vi "Aux CO2 Serial Close.vi"(8 "error in":errorcluster, 10 "Capno Data In":T1={"Port"="", "Source"=0, "Active"=FALSE, "Baro Pressure"=760, "SerialRxBuffer"="", "Raw CO2 (Torr)"=5.0, "bytes read"=5, "Status"=[], "Status Message"=enum.""} {"Status" format="%x"; "Baro Pressure" min=400 max=800; "Source" items=["None", "TidalWave", "LoFlow / Canary", "Capnogard"]}, 11 "Serial Port In":T3={"termination char"=10, "End read on termination character?"=TRUE, "Enabled?"=FALSE, "VISA resource name"="COM1", "baud rate"=9600, "data bits"=8, "parity"=enum."None", "stop bits"=10, "flow control"=0, "timeout (ms)"=10000, "Input buffer size"=4096, "End write on termination character?"=TRUE, "XON Char"=17, "XOFF Char"=19} {"XOFF Char" format="%.0x"; "XON Char" format="%.0x"; "flow control" items=["None"=0, "XON/XOFF"=1, "RTS/CTS"=2, "DTR/DSR"=4]; "stop bits" items=["1.0"=10, "1.5"=15, "2.0"=20]; "data bits" min=5 max=8 step=1; "baud rate" items=["75"=75, "110"=110, "134"=134, "150"=150, "300"=300, "600"=600, "1200"=1200, "1800"=1800, "2400"=2400, "4800"=4800, "7200"=7200, "9600"=9600, "14400"=14400, "19200"=19200, "28800"=28800, "38400"=38400, "56000"=56000, "57600"=57600, "115200"=115200, "128000"=128000, "230400"=230400]; "termination char" format="%.0x"}) -> (0 "error out":errorcluster, 2 "Capno Data Out":T1={"Port"="", "Source"=0, "Active"=FALSE, "Baro Pressure"=760, "SerialRxBuffer"="", "Raw CO2 (Torr)"=5.0, "bytes read"=5, "Status"=[], "Status Message"=enum.""} {"Status" format="%x"; "Baro Pressure" min=400 max=800; "Source" items=["None", "TidalWave", "LoFlow / Canary", "Capnogard"]}, 3 "Serial Port Out":T3={"termination char"=10, "End read on termination character?"=TRUE, "Enabled?"=TRUE, "VISA resource name"="COM1", "baud rate"=9600, "data bits"=8, "parity"=enum."None", "stop bits"=10, "flow control"=0, "timeout (ms)"=10000, "Input buffer size"=4096, "End write on termination character?"=FALSE, "XON Char"=17, "XOFF Char"=19} {"XOFF Char" format="%.0x"; "XON Char" format="%.0x"; "flow control" items=["None"=0, "XON/XOFF"=1, "RTS/CTS"=2, "DTR/DSR"=4]; "stop bits" items=["1.0"=10, "1.5"=15, "2.0"=20]; "baud rate" items=["1.0"=10, "1.5"=15, "2.0"=20]; "termination char" format="%.0x"})   [LabVIEW 2016]
uses:
  Controls/Serial Visa Control.ctl
  Controls/Aux CO2 Diags.ctl
  Controls/Aux CO2 Selector.ctl
  Controls/SerialPortControl.ctl
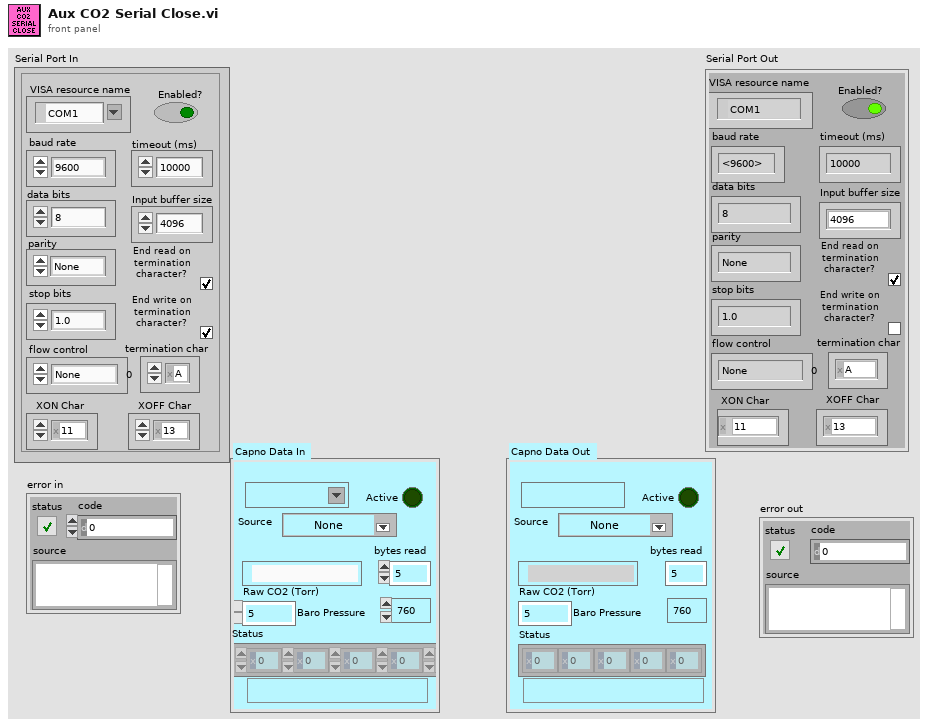
[diagram p1: front panel]
types:
  T1 = typedef "Aux CO2 Diags.ctl" = cluster{"Port":refnum<visa-resource-name>, "Source":T2, "Active":bool, "Baro Pressure":u16, "SerialRxBuffer":string, "Raw CO2 (Torr)":sgl, "bytes read":i16, "Status":u8[], "Status Message":enum16{"", "Sensor Over Temp", "Sensor Faulty", "Set BaroP", "Capno in Sleep Mode", "Zero In Progress", "Sensor Warm Up", "Check Sampling Line", "Zero Required", "CO2 Out Of Range", "Check Airway Adapter", "LoFlo Not Connected"}}
  T2 = typedef "Aux CO2 Selector.ctl" = u16
  T3 = typedef "Serial Visa Control.ctl" = cluster{"termination char":u8, "End read on termination character?":bool, "Enabled?":bool, "VISA resource name":refnum<visa-resource-name>, "baud rate":u32, "data bits":u16, "parity":enum16{"None", "Odd", "Even", "Mark", "Space"}, "stop bits":u16, "flow control":u16, "timeout (ms)":u32, "Input buffer size":u32, "End write on termination character?":bool, "XON Char":u8, "XOFF Char":u8}
  T4 = typedef "SerialPortControl.ctl" = enum16{"Initialize", "Write Data", "Read Data", "Close Port"}
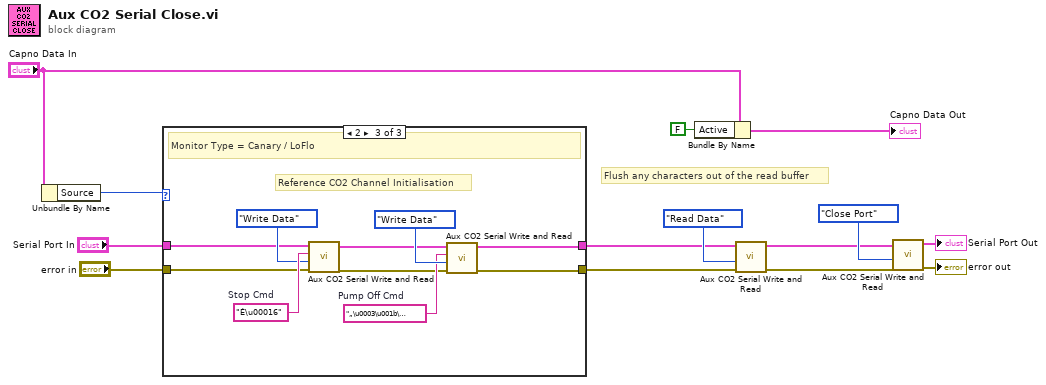
[diagram p0: block diagram]
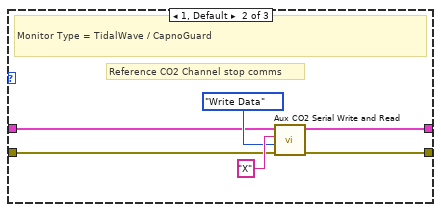
[diagram p3: hidden frame]
diagram:
  # "Flush any characters out of the read buffer"
  n1 = Unbundle By Name("Capno Data In") -> ("Source"=w4:T2)
  n2 = case shown="2" w4 {
    tunnel: "Serial Port In" -> [w16 w17 w30]
    tunnel: [w15 w19 w24] -> w10
    tunnel: "error in" -> [w15 w18 w29]
    tunnel: [w16 w20 w23] -> w9
    frame 0 {
      # "Monitor Type = None"
    }
    frame 1, Default {
      # "Reference CO2 Channel stop comms"
      # "Monitor Type = TidalWave / CapnoGuard"
      n3 = call "Aux CO2 Serial Write and Read.vi"("error in"=w18, "Action"=SerialPortControl."Write Data", "string to write"="X", "Serial Port"=w17) -> ("error IO"=w19:errorcluster, "Serial Port Out"=w20:T3)  [unwired: 2 out]
    }
    frame 2 {
      w27 = "„\u0003\u001b\u0001]"  # Pump Off Cmd
      w32 = "É\u00016"  # Stop Cmd
      # "Reference CO2 Channel Initialisation"
      # "Monitor Type = Canary / LoFlo"
      n4 = call "Aux CO2 Serial Write and Read.vi"("error in"=w29, "Action"=SerialPortControl."Write Data", "string to write"=w32, "Serial Port"=w30) -> ("error IO"=w26:errorcluster, "Serial Port Out"=w25:T3)  [unwired: 2 out]
      n5 = call "Aux CO2 Serial Write and Read.vi"("error in"=w26, "Action"=SerialPortControl."Write Data", "string to write"=w27, "Serial Port"=w25) -> ("error IO"=w24:errorcluster, "Serial Port Out"=w23:T3)  [unwired: 2 out]
    }
  }
  n6 = Bundle By Name(cluster="Capno Data In", "Active"=FALSE) -> (→"Capno Data Out":T1)
  n7 = call "Aux CO2 Serial Write and Read.vi"("error in"=w10, "Action"=SerialPortControl."Read Data", "Serial Port"=w9) -> ("error IO"=w11:errorcluster, "Serial Port Out"=w12:T3)  [unwired: 1 in, 2 out]
  n8 = call "Aux CO2 Serial Write and Read.vi"("error in"=w11, "Action"=SerialPortControl."Close Port", "Serial Port"=w12) -> ("error IO"=→"error out":errorcluster, "Serial Port Out"=→"Serial Port Out":T3)  [unwired: 1 in, 2 out]
